vi "getZsuffix.vi"(6 "format string":string="%02d", 7 "label":string="z", 9 "Units":string="um", 11 "Zposition":dbl) -> (3 "String":string="z00um")   [LabVIEW 2023]
panel:
  # "%03d -> integer 0 padded to be at least 3 digits\n\n%05.2f -> float with 2 decimals and 0 padded \n                  to be at least 5 digits (including all, also the point)"
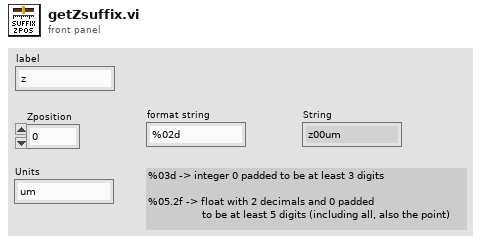
[diagram p1: front panel]
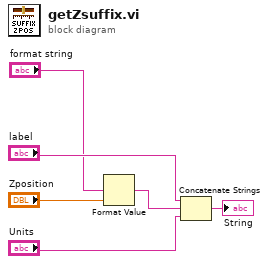
[diagram p0: block diagram]
diagram:
  n1 = Format Value(format string="format string", value (0)="Zposition") -> (output string=w3:string)  [unwired: 1 in]
  n2 = Concatenate Strings("label", w3, "Units") -> (→"String":string)
